vi "Do Something.vi"(8 "error in (no error)":errorcluster, 10 "Do Something Message":string, 11 "TemplateAPI in":refnum<class "ExampleAPI.lvclass">) -> (0 "error out":errorcluster, 3 "TemplateAPI out":refnum<class "ExampleAPI.lvclass">)   [LabVIEW 2018, in "ExampleAPI.lvclass"]
uses:
  ExampleAPI.lvclass
  C:/Users/Phalanx/Documents/LabVIEW-Application-API-Template/src/Classes/AppControlAPI/AppControlAPI.lvclass
  AppControlAPI/AppControlAPI.lvclass/AppControlAPI.ctl
  4c94efee-2ba9-4b86-bf77-9303cd5a5534.vi
  AppControlAPI/Read AppRef.vi
  AppControlAPI/Insert In Reference Cache.vi
  AppControlAPI/Read Cache.vi
  AppControlAPI/Write Cache.vi
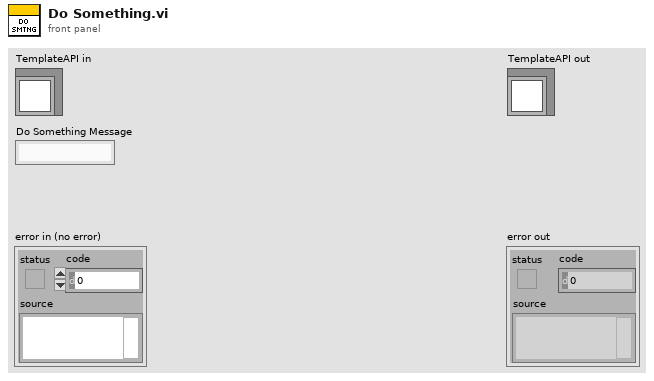
[diagram p1: front panel]
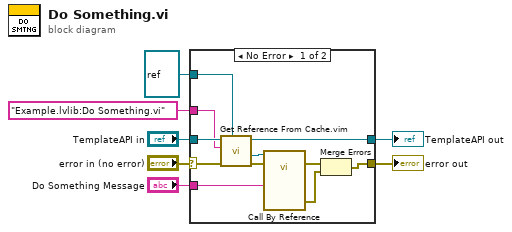
[diagram p0: block diagram]
diagram:
  n1 = case shown="No Error" "error in (no error)" {
    selector: "error in (no error)" -> [w14 w20]
    tunnel: [w11 w20] -> w6
    tunnel: [w17 w19] -> w4
    tunnel: "TemplateAPI in" -> [w18 w19]
    tunnel: "Do Something Message" -> [w12 _]
    tunnel: "Example.lvlib:Do Something.vi" ("VIQualifiedName") -> [w9 _]
    tunnel: refnum<vi> refnum ("type specifier VI Refnum (for type only)") -> [w8 _]
    frame No Error {
      n2 = call "Get Reference From Cache.vim"("type specifier VI Refnum (for type only)"=w8, "error in (no error)"=w14, "VIQualifiedName"=w9, "AppControlAPI in"=w18) -> ("error out"=w15:errorcluster, "VIRef"=w16:refnum<vi>, "AppControlAPI out"=w17:refnum<class "ExampleAPI.lvclass">)  [unwired: 5 in]
      n3 = call-by-ref "?"(reference=w16, error in=w15, "Do Something Message"=w12) -> (error out=w13:errorcluster, 0:"error out"=w10:errorcluster)  [unwired: 10 in, 1 out]
      n4 = Merge Errors(w13, w10) -> (w11:errorcluster)
    }
    frame Error {
    }
  }
  "error out" <- w6
  "TemplateAPI out" <- w4
